vi "Practica 3.vi"() -> ()   [LabVIEW 2018]
uses:
  <vilib>/express/express analysis/Spectral/Block/exnSpectralBlock spectral measurements RMS poly.vi
  <vilib>/express/express analysis/Spectral/Block/exnSpectralBlock spectral measurements RMS DDT.vi
  <vilib>/express/express analysis/Spectral/XNode/ExpressSpectralMeasurementsBlockNode.xnode
panel:
  out "Grafica de la senal 1 en el dominio de la frecuencia":dynamicdata(graph)
  out "Grafica de la senal 1 en el dominio del tiempo":dynamicdata(graph)
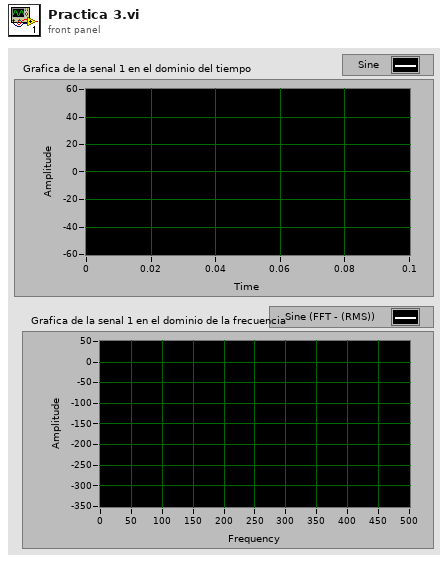
[diagram p1: front panel]
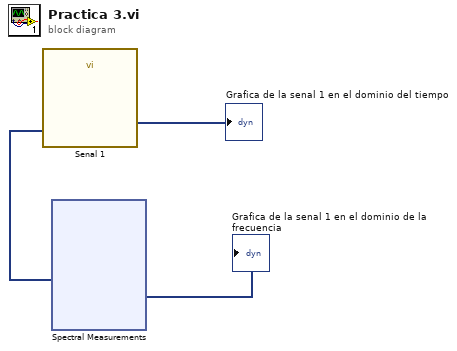
[diagram p0: block diagram]
diagram:
  n1 = call "Senal 1"() -> ("Sine"=w1:dynamicdata)  [unwired: 14 in, 1 out]
  "Grafica de la senal 1 en el dominio del tiempo" <- w1
  n2 = xnode "Spectral Measurements"("Signals"=w1) -> ("FFT - (RMS)"=→"Grafica de la senal 1 en el dominio de la frecuencia":dynamicdata)  [unwired: 1 in, 2 out]
